vi "initialize scope.vi"(4 "error in":errorcluster, 7 "resource name":refnum<k15>) -> (0 "error out":errorcluster, 1 "Self-test complete":bool, 2 "Scope on":bool, 3 "instrument handle":refnum<k15> caption="Scope Resource Name Out")   [LabVIEW 2018]
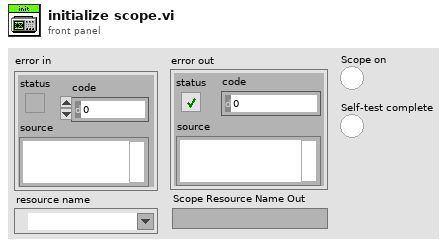
[diagram p1: front panel]
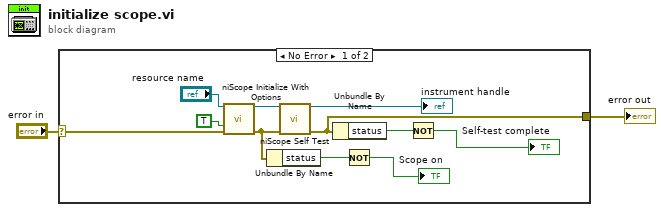
[diagram p0: block diagram]
diagram:
  n1 = case shown="No Error" "error in" {
    selector: "error in" -> [w6 w14]
    tunnel: [w3 w14] -> w2
    frame No Error {
      n2 = call <instrlib>:"niScope Initialize With Options.vi"("resource name"="resource name", "reset device"=TRUE, "error in"=w6) -> ("instrument handle"=w13:refnum<k15>, "error out"=w9:errorcluster)  [unwired: 2 in, 9 out]
      n3 = Unbundle By Name(w9) -> ("status"=w10:bool)
      n4 = call <instrlib>:"niScope Self Test.vi"("instrument handle"=w13, "error in"=w9) -> ("instrument handle out"=→"instrument handle":refnum<k15>, "error out"=w3:errorcluster)  [unwired: 10 in, 2 out]
      n5 = Unbundle By Name(w3) -> ("status"=w4:bool)
      n6 = Not(x=w10) -> (.not. x?=→"Scope on":bool)
      n7 = Not(x=w4) -> (.not. x?=→"Self-test complete":bool)
    }
    frame Error {
    }
  }
  "error out" <- w2
